vi "压电.vi"() -> ()   [LabVIEW 2010]
doc: "Cont(inuous) Acq(uire) & Graph (buffered) demonstrates buffered data acquisition. Data is continuously acquired into a circular buffer at the same time that data previously retrieved from the buffer is plotted. This VI also demonstrates how to plot multiple points from multiple channels on a graph. \n\nBefore running this VI, set the values of the controls on the front panel. Select Show Help Window from the Help menu to see a description of each control. If the values you select for all the controls are values you will usually use, select Make Current Values Default from the Operate menu and save the VI. Or, you may save individual control's default values by popping up on the control, selecting Data Operations, then selecting Make Current Value Default, and saving the VI.\n\n\nThe buffer size is the number of scans that will be held in the internal memory buffer, and is limited by the amount of memory available. Experiment with the buffer size and the number of scans to read each time. If the buffer is too small or you are not reading data from it fast enough, your data will be overwritten by new data before you have a chance to read it (overwrite error). If the buffer is too big, you will run out of memory (out of memory error).\n\n\nYou will probably want to add more functions to the diagram to customize this VI for your application. A common reason to read data while the acquisition is in progress is to process and display the data in pseudo-real time. The acquisition rate you can achieve depends on how much processing and display the VI must do. This VI calls a subVI named My Data Processing. Add whatever processing you need to this subVI, or replace it with one of your own. The data processing subVI also demonstrates how to use error clusters in your own subVIs, so they can be included in the error data flow chain."
panel:
  in  "stop":bool
  out "力值（N）":dbl[](graph) caption="waveform graph"
  # "测力传感器实验"
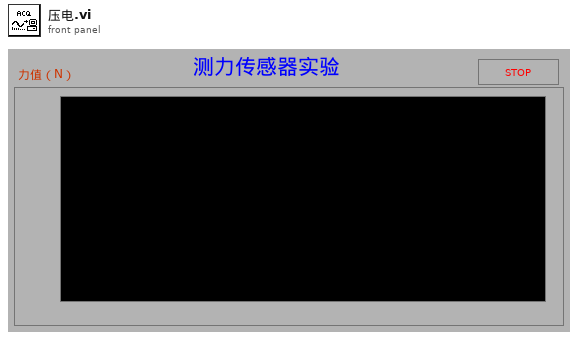
[diagram p1: front panel]
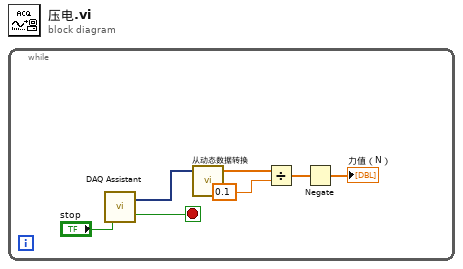
[diagram p0: block diagram]
diagram:
  n1 = while {
    stop <- w7 stop-if-true
    n2 = call "DAQ Assistant"("stop (F)"="stop") -> ("data"=w4:dynamicdata, "stopped"=w7:bool)  [unwired: 15 in, 2 out]
    n3 = call "从动态数据转换"("Dynamic Data Type"=w4) -> ("Array"=w3:dbl[])  [unwired: 3 in]
    n4 = Divide(x=w3, y=0.1) -> (x/y=w5:dbl[])
    n5 = Negate(x=w5) -> (-x=→"力值（N）":dbl[])
  }
